vi "Has Next.vi"(8 "error in (no error)":errorcluster, 11 "Continuous.lvclass in":refnum<class "Continuous.lvclass">) -> (0 "error out":errorcluster, 2 "Again?":bool, 3 "Continuous.lvclass out":refnum<class "Continuous.lvclass">)   [LabVIEW 2009, in "Continuous.lvclass"]
uses:
  Continuous.lvclass
  Scanner/Scanner.lvclass
  Instruments/Magnet/Magnet.lvclass
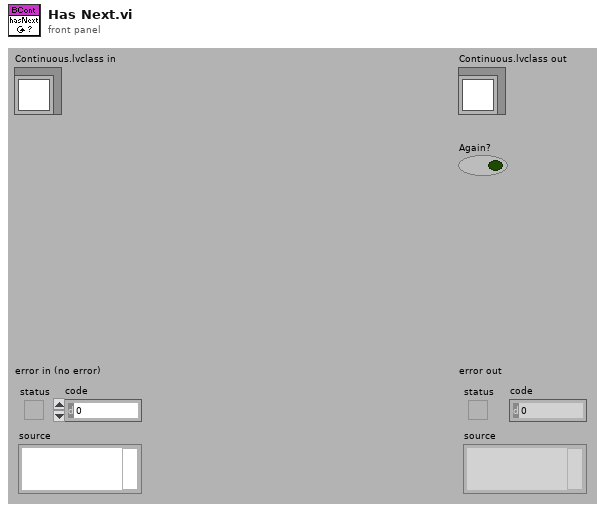
[diagram p1: front panel]
types:
  T1 = typedef "Scanner.lvclass/Range.ctl" = cluster{"xi":dbl, "xf":dbl, "dx":dbl, "Return to start?":bool}
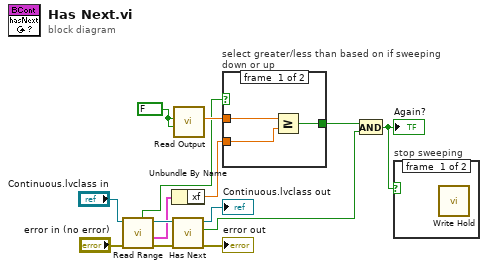
[diagram p0: block diagram]
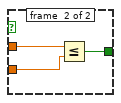
[diagram p2: hidden frame]
diagram:
  w11 = FALSE
  n1 = call-dynamic "Read Range.vi"("error in (no error)"="error in (no error)", "Scanner.lvclass in"="Continuous.lvclass in") -> ("error out"=w3:errorcluster, "Range"=w8:T1, "Scanner.lvclass out"=w12:refnum<class "Continuous.lvclass">, "Scanning Up?"=w2:bool)  [unwired: 6 out]
  n2 = Unbundle By Name(w8) -> ("xf"=w1:dbl)
  n3 = call-parent "Has Next.vi"("error in (no error)"=w3, "Scanner.lvclass in"=w12) -> ("error out"=→"error out":errorcluster, "Again?"=w6:bool, "Scanner.lvclass out"=→"Continuous.lvclass out":refnum<class "Continuous.lvclass">)  [unwired: 7 out]
  n4 = call "Read Output.vi"("checkpers?"=w11, "amp?"=w11) -> ("ouput"=w10:dbl)  [unwired: 5 out]
  n5 = case "select greater/less than based on if sweeping down or up" shown="True" w2 {
    tunnel: w10 -> [w17 w19]
    tunnel: w1 -> [w16 w20]
    tunnel: [w15 w18] -> w7
    frame #0 {
      n6 = Greater Or Equal?(x=w17, y=w16) -> (x >= y?=w15:bool)
    }
    frame #1 {
      n7 = Less Or Equal?(x=w19, y=w20) -> (x <= y?=w18:bool)
    }
  }
  n8 = And(x=w7, y=w6) -> (x .and. y?=w5:bool)
  "Again?" <- w5
  n9 = case "stop sweeping" shown="False" w5 {
    frame #0 {
      n10 = call "Write Hold.vi"() -> ()  [unwired: 8 out]
    }
    frame #1 {
    }
  }
